vi "Obtain Group.vi"(7 "Group Type (Abstract)":refnum<class "Group.lvclass">, 8 "error in (no error)":errorcluster, 9 "Timeout ms (5000)":u32=5000, 10 "Group Name":string, 11 "VolatusAPI in":refnum<class "VolatusAPI.lvclass">) -> (0 "error out":errorcluster, 2 "Group":refnum<class "Group.lvclass">, 3 "VolatusAPI out":refnum<class "VolatusAPI.lvclass">)   [LabVIEW 2020, in "Volatus.lvlib" / "VolatusAPI.lvclass"]
uses:
  VolatusAPI.lvclass
  lv-vecto/Vecto/Group/Group.lvclass
  VolatusConfig/Meta Type.ctl
  VolatusAPI.lvclass/VolatusAPI.ctl
  VolatusConfig/VolatusConfigElement/VolatusConfigElement.lvclass/VolatusConfigElement.ctl
  25fe4c30-a09b-47ff-bb6b-02640d7dd0a1.vi
  VolatusConfig/VolatusConfigElement/Element.vi
  VolatusConfig/Node/Node Config.lvclass
  C:/dev/lv20CE/relink/lv-volatus/VolatusConfig/VolatusConfigElement/VolatusConfigElement.lvclass
  lv-cdm/CDM-Config/Config Lookup/Match Meta.vi
  lv-cdm/CDM-Config/Config Element/Owner.vi
  lv-cdm/CDM-Config/Config Manager/Lookup Descendant.vi
  lv-cdm/CDM-Config/Config Filter/Config Lookup.lvclass
  VolatusConfig/VolatusConfigElement/VolatusConfigElement.lvclass
  VolatusConfig/VolatusConfig.lvlib
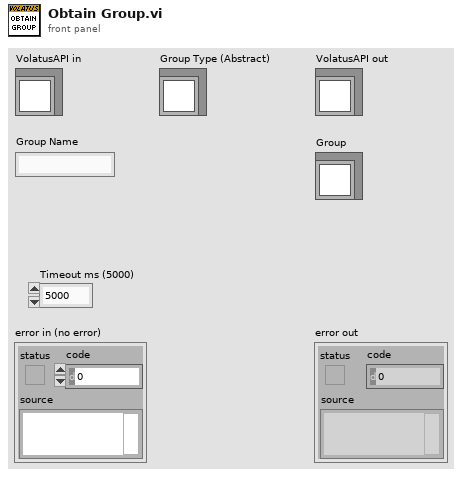
[diagram p1: front panel]
types:
  T1 = typedef "VolatusConfig.lvlib/Meta Type.ctl" = enum16{"UNKNOWN", "VL_System", "VL_Cluster", "VL_Node", "VL_Task", "VL_Group", "VL_Channel", "VL_Task_List", "VL_Scaling", "VL_Sensor", "VL_Sensor_List", "VL_Scale"}
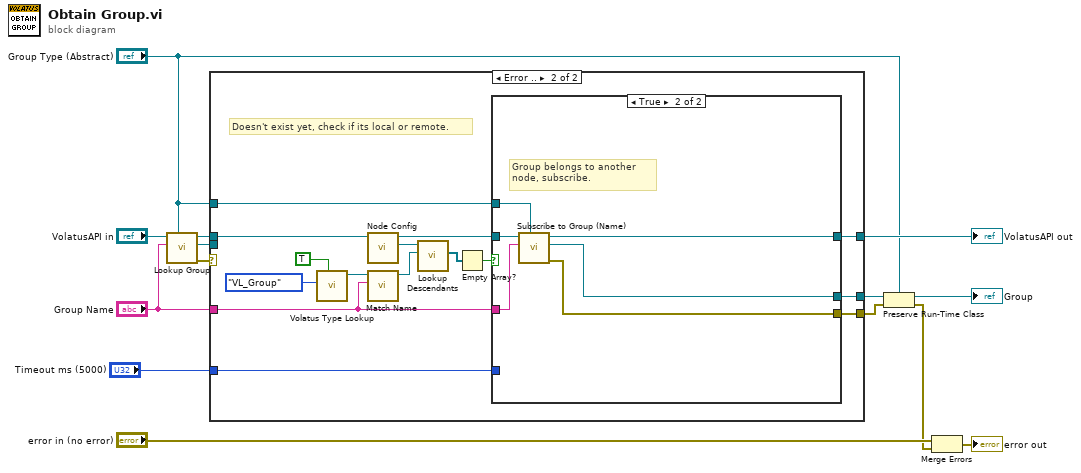
[diagram p0: block diagram]
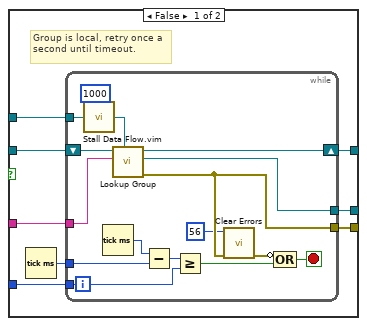
[diagram p3: hidden frame]
diagram:
  n1 = call "Lookup Group.vi"("Group Type (Abstract)"="Group Type (Abstract)", "Group Name"="Group Name", "VolatusAPI in"="VolatusAPI in") -> ("error out"=w12:errorcluster, "Group"=w11:refnum<class "Group.lvclass">, "VolatusAPI out"=w8:refnum<class "VolatusAPI.lvclass">)  [unwired: 6 in]
  n2 = case shown="Error .." w12 {
    tunnel: w11 -> [w16 _]
    tunnel: [w16 w19] -> w10
    tunnel: [w15 w20] -> w9
    tunnel: w8 -> [w15 w31]
    tunnel: "Group Name" -> [_ w21]
    tunnel: "Group Type (Abstract)" -> [_ w22]
    tunnel: [_ w18] -> w4
    tunnel: "Timeout ms (5000)" -> [_ w17]
    frame No Error {
    }
    frame Error {
      # "Doesn't exist yet, check if its local or remote."
      n3 = call "Volatus Type Lookup.vi"("Don't Recurse Past Match (F)"=TRUE, "Meta Type"=Meta_Type."VL_Group") -> ("Config Lookup out"=w28:refnum<class "Config Lookup.lvclass">)  [unwired: 8 in, 1 out]
      n4 = call "Node Config.vi"("VolatusAPI in"=w31) -> ("Node Config"=w30:refnum<class "Node Config.lvclass">, "VolatusAPI out"=w23:refnum<class "VolatusAPI.lvclass">)  [unwired: 9 in]
      n5 = call "Match Name.vi"("Name"=w21, "Config Lookup (New)"=w28) -> ("Config Lookup out"=w26:refnum<class "Config Lookup.lvclass">)  [unwired: 8 in, 1 out]
      n6 = call "Lookup Descendants.vi"("Lookup"=w26, "VolatusConfigElement in"=w30) -> ("Descendants"=w25:refnum<class "Config Element.lvclass">[])  [unwired: 7 in, 2 out]
      n7 = Empty Array?(array=w25) -> (empty?=w24:bool)
      n8 = case shown="True" w24 {
        tunnel: w23 -> [w35 w61]
        tunnel: w22 -> [w39 w60]
        tunnel: w21 -> [w36 w59]
        tunnel: [w32 w58] -> w20
        tunnel: [w33 w57] -> w19
        tunnel: [w34 w56] -> w18
        tunnel: w17 -> [w37 _]
        frame False {
          # "Group is local, retry once a second until timeout."
          n9 = Tick Count (ms)() -> (millisecond timer value=w38:u32)
          n10 = while {
            tunnel: w39 -> [w52]
            tunnel: w38 -> [w55]
            tunnel: w37 -> [w47]
            tunnel: w36 -> [w49]
            tunnel: [w41] -> w34
            tunnel: [w44] -> w33
            shift-right: [w43] -> w32
            shift-left: w35 -> [w53]
            stop <- w45 stop-if-true
            n11 = call "Stall Data Flow.vim"("value in"=w52, "milliseconds to wait"=u32 1000) -> ("value out"=w51:refnum<class "Group.lvclass">)  [unwired: 1 out]
            n12 = Tick Count (ms)() -> (millisecond timer value=w54:u32)
            n13 = call "Lookup Group.vi"("Group Type (Abstract)"=w51, "Group Name"=w49, "VolatusAPI in"=w53) -> ("error out"=w41:errorcluster, "Group"=w44:refnum<class "Group.lvclass">, "VolatusAPI out"=w43:refnum<class "VolatusAPI.lvclass">)  [unwired: 6 in]
            n14 = Subtract(x=w54, y=w55) -> (x-y=w48:u32)
            n15 = Greater Or Equal?(x=w48, y=w47) -> (x >= y?=w46:bool)
            n16 = call <vilib>:"Clear Errors.vi"("error in (no error)"=w41, "specific error code to clear (0: all)"=56) -> ("error out"=w42:errorcluster)  [unwired: 4 in, 1 out]
            n17 = Compound Arithmetic op=OR(invert w42, w46) -> (w45:bool)
          }
        }
        frame True {
          # "Group belongs to another node, subscribe."
          n18 = call "Subscribe to Group (Name).vi"("Group Type"=w60, "Group Name"=w59, "VolatusAPI in"=w61) -> ("error out"=w56:errorcluster, "Group"=w57:refnum<class "Group.lvclass">, "VolatusAPI out"=w58:refnum<class "VolatusAPI.lvclass">)  [unwired: 6 in]
        }
      }
    }
  }
  "VolatusAPI out" <- w9
  n19 = Preserve Run-Time Class(object in=w10, error in=w4, 2:"Group Type (Abstract)") -> (object out=→"Group":refnum<class "Group.lvclass">, error out=w2:errorcluster)
  n20 = Merge Errors("error in (no error)", w2) -> (→"error out":errorcluster)
